vi "RefreshTafMenu.vi"(8 "ErrorIn":errorcluster, 11 "ObjectIn":refnum<class "MasterGUI.lvclass">) -> (0 "ErrorOut":errorcluster, 3 "ObjectOut":refnum<class "MasterGUI.lvclass">)   [LabVIEW 2021, in "MasterGUI.lvclass"]
uses:
  MasterGUI.lvclass
  MasterGUI.lvclass/MasterGUI.ctl
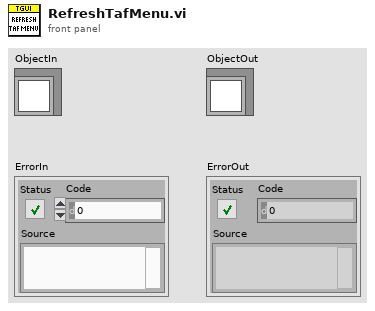
[diagram p1: front panel]
types:
  T1 = typedef "MasterGUI.lvclass/ObjectAttributes.ctl" = cluster{"Interfaces":cluster{"Dummy":refnum<class>}, "Locals":cluster{"MainGUIActive":refnum<queue>, "MainPanel":refnum<vi>, "LayoutPanel":cluster{"PanelVIRef":refnum<vi>, "Labels":string[], "SubPanels":refnum<vi>[]}, "MenuTree":T2[], "Menu":refnum<k9>}, "Persistent":cluster{"StaticDocking":cluster{"ObjectLabel":string, "SubPanelLabel":string}[], "WindowsTitle":string, "AdditionalMenuItems":T2[], "TraceObjectName":string}}
  T2 = typedef "MasterGUI.lvclass/MenuItem.ctl" = cluster{"Parent":string, "Items":string[], "ShortCuts":cluster{"IncludeShiftKey":bool, "IncludeCtrlKey":bool, "ShortcutKey":string}[]}
  T3 = cluster{"IncludeShiftKey":bool, "IncludeCtrlKey":bool, "ShortcutKey":string}[]
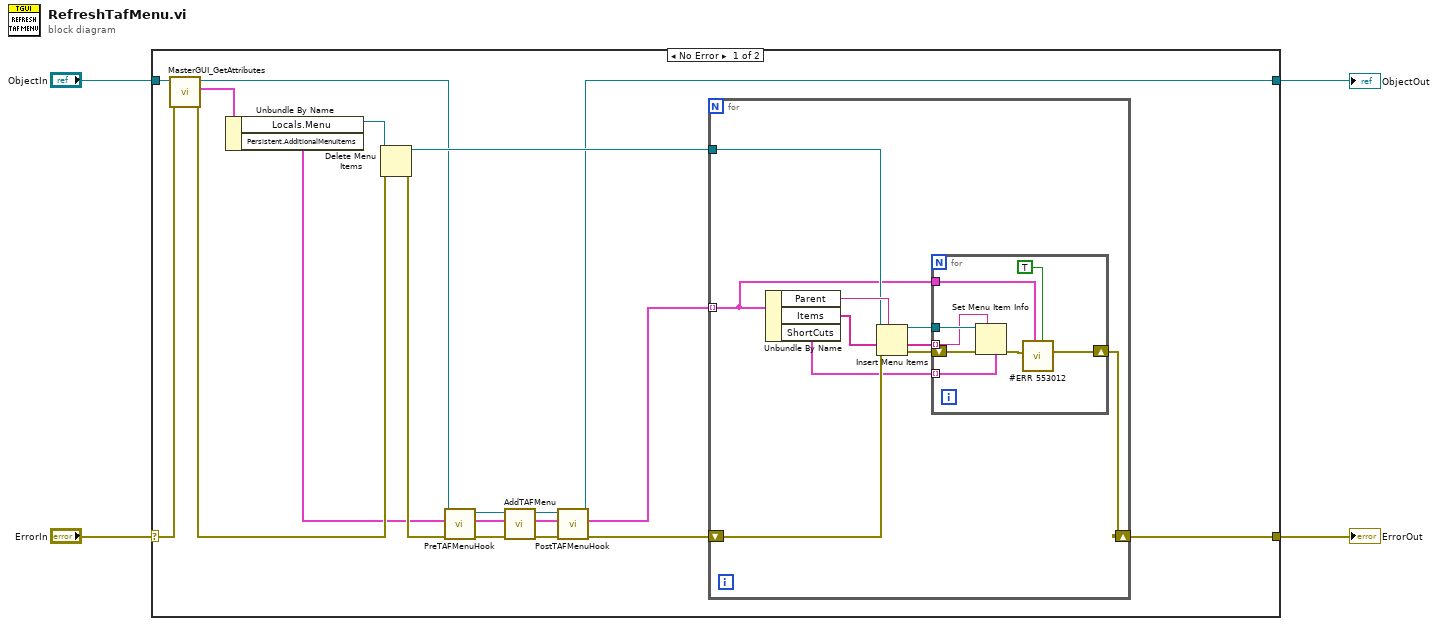
[diagram p0: block diagram]
diagram:
  n1 = case shown="No Error" "ErrorIn" {
    selector: "ErrorIn" -> [w21 w43]
    tunnel: [w17 w43] -> w4
    tunnel: [w5 w42] -> w1
    tunnel: "ObjectIn" -> [w16 w42]
    frame No Error {
      n2 = call "MasterGUI_GetAttributes.vi"("error in (no error)"=w21, "reference in"=w16) -> ("error out"=w20:errorcluster, "Data"=w15:T1, "reference out"=w7:refnum<class "MasterGUI.lvclass">)  [unwired: 6 in, 1 out]
      n3 = Unbundle By Name(w15) -> ("Locals.Menu"=w14:refnum<k9>, "Persistent.AdditionalMenuItems"=w6:T2[])
      n4 = Delete Menu Items(6:w20, 9:w14) -> (0:w23:errorcluster, 3:w13:refnum<k9>)  [unwired: 2 in]
      n5 = call-dynamic "PreTAFMenuHook.vi"("error in (no error)"=w23, "MenuIn"=w6, "MasterGUI in"=w7) -> ("error out"=w19:errorcluster, "MenuOut"=w12:T2[], "MasterGUI out"=w11:refnum<class "MasterGUI.lvclass">)  [unwired: 6 in]
      n6 = call-dynamic "AddTAFMenu.vi"("error in (no error)"=w19, "MenuIn"=w12, "MasterGUI in"=w11) -> ("error out"=w22:errorcluster, "MenuOut"=w8:T2[], "MasterGUI out"=w10:refnum<class "MasterGUI.lvclass">)  [unwired: 6 in]
      n7 = call-dynamic "PostTAFMenuHook.vi"("error in (no error)"=w22, "MenuIn"=w8, "MasterGUI in"=w10) -> ("error out"=w18:errorcluster, "MenuOut"=w9:T2[], "MasterGUI out"=w5:refnum<class "MasterGUI.lvclass">)  [unwired: 6 in]
      n8 = for {
        tunnel: w9 -> [w24] mode=indexing
        shift-right: [w31] -> w17
        shift-left: w18 -> [w33]
        tunnel: w13 -> [w28]
        n9 = Unbundle By Name(w24) -> ("Parent"=w29:string, "Items"=w30:string[], "ShortCuts"=w25:T3)
        n10 = Insert Menu Items(5:w29, 6:w33, 7:w30, 9:w28) -> (0:w32:errorcluster, 1:w26:string[], 3:w27:refnum<k9>)  [unwired: 2 in]
        n11 = for {
          tunnel: w27 -> [w38]
          shift-right: [w39] -> w31
          shift-left: w32 -> [w41]
          tunnel: w26 -> [w37] mode=indexing
          tunnel: w25 -> [w36] mode=indexing
          tunnel: w24 -> [w35]
          n12 = Set Menu Item Info(4:w36, 7:w37, 8:w41, 11:w38) -> (0:w40:errorcluster)  [unwired: 3 in, 1 out]
          n13 = call "#ERR 553012"("MergeErrors"=TRUE, "Data"=w35, "error in (no error)"=w40) -> ("error out"=w39:errorcluster)  [unwired: 8 in]
        }
      }
    }
    frame Error {
    }
  }
  "ErrorOut" <- w4
  "ObjectOut" <- w1
